vi "Send I32 Value.vi"(6 "Name (use label text)":string, 8 "error in (no error)":errorcluster, 9 "Value":i32, 10 "I32 Refnum":refnum<vi>, 11 "Message Enqueuer in":refnum<class "Message Enqueuer.lvclass">) -> (0 "error out":errorcluster)   [LabVIEW 2015, in "ActorAutoRegistration.lvlib" / "I32ValueMsg.lvclass"]
uses:
  I32ValueMsg.lvclass
  <vilib>/ActorFramework/Message Enqueuer/Message Enqueuer.lvclass
  I32ValueMsg.lvclass/I32ValueMsg.ctl
  EventDataMessage/EventDataMessage.lvclass
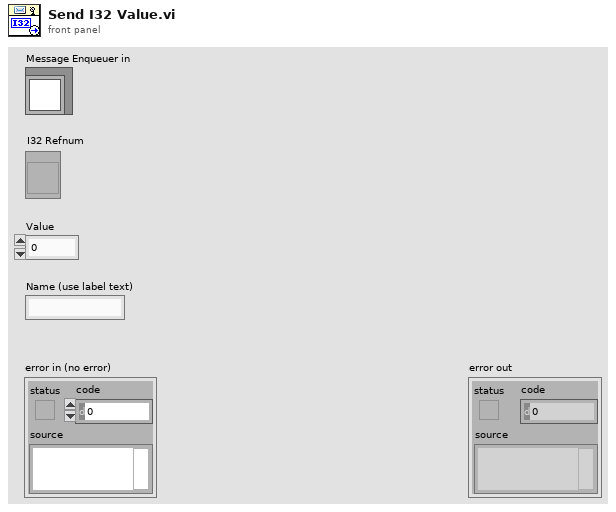
[diagram p1: front panel]
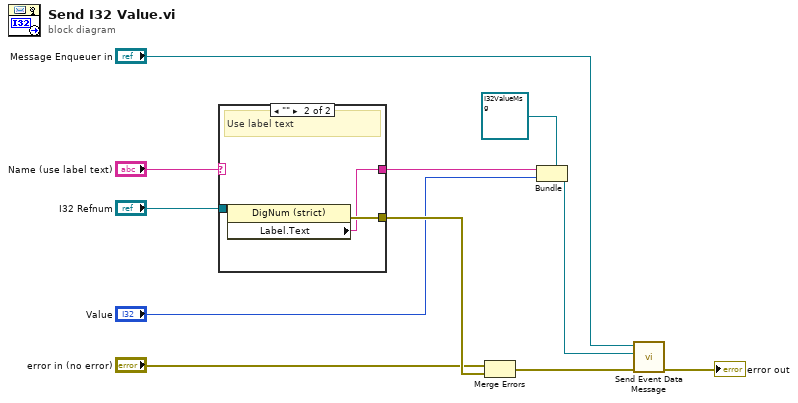
[diagram p0: block diagram]
diagram:
  n1 = case shown="\"\"" "Name (use label text)" {
    selector: "Name (use label text)" -> [w12 _]
    tunnel: [w12 w13] -> w11
    tunnel: "I32 Refnum" -> [_ w15]
    tunnel: [_ w14] -> w9
    frame Default {
      # "Use string provided"
    }
    frame "" {
      # "Use label text"
      n2 = property class="DigNum (strict)"(reference=w15) -> (error out=w14:errorcluster, "Label.Text"=w13:string)  [unwired: 1 in, 1 out]
    }
  }
  n3 = Merge Errors("error in (no error)", w9) -> (w10:errorcluster)
  n4 = Bundle(cluster=refnum<class "I32ValueMsg.lvclass"> refnum ("I32ValueMsg"), w11, "Value") -> (w8:refnum<class "I32ValueMsg.lvclass">)
  n5 = call "Send Event Data Message.vi"("error in (no error)"=w10, "EventDataMessage in"=w8, "Message Enqueuer in"="Message Enqueuer in") -> ("error out"=→"error out":errorcluster)  [unwired: 8 in]
